vi "laserDiagnose.vi"(0 "405 Port":refnum<visa-resource-name>, 1 "ms to wait (50)":u32=50, 5 "532 Port":refnum<visa-resource-name>, 7 "660 Port":refnum<visa-resource-name>, 9 "785 Port":refnum<visa-resource-name>, 11 "error in (no error)":errorcluster) -> (4 "Currents":T1, 6 "Temperatures":T2, 10 "Powers":T3, 14 "Overtemp":bool, 15 "error out":errorcluster)   [LabVIEW 2011]
panel:
  out "660 Port Out":refnum<visa-resource-name>
  out "532 Port Out":refnum<visa-resource-name>
  out "405 Port Out":refnum<visa-resource-name>
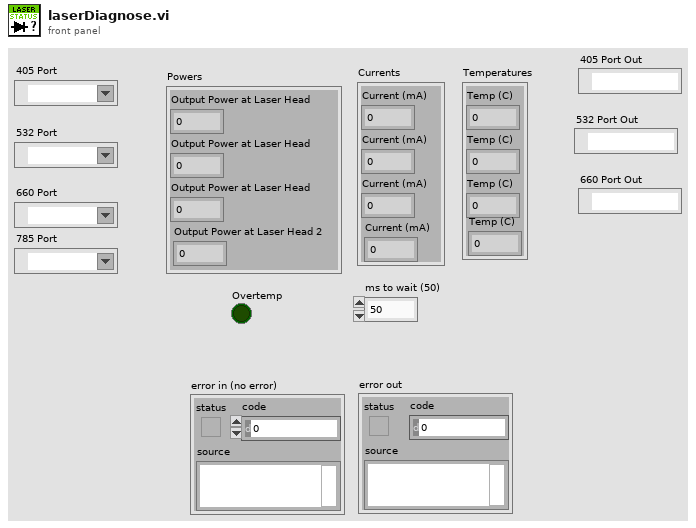
[diagram p1: front panel]
types:
  T1 = cluster{"Current (mA)":dbl, "Current (mA)":dbl, "Current (mA)":dbl, "Current (mA)":dbl}
  T2 = cluster{"Temp (C)":dbl, "Temp (C)":dbl, "Temp (C)":dbl, "Temp (C)":dbl}
  T3 = cluster{"Output Power at Laser Head":dbl, "Output Power at Laser Head":dbl, "Output Power at Laser Head":dbl, "Output Power at Laser Head 2":dbl}
  T4 = cluster{"Current, mA":dbl, "Current, mA":dbl, "Current, mA":dbl, "Current, mA":dbl}
  T5 = cluster{"Power, mW":dbl, "Power, mW":dbl, "Power, mW":dbl, "Power, mW":dbl}
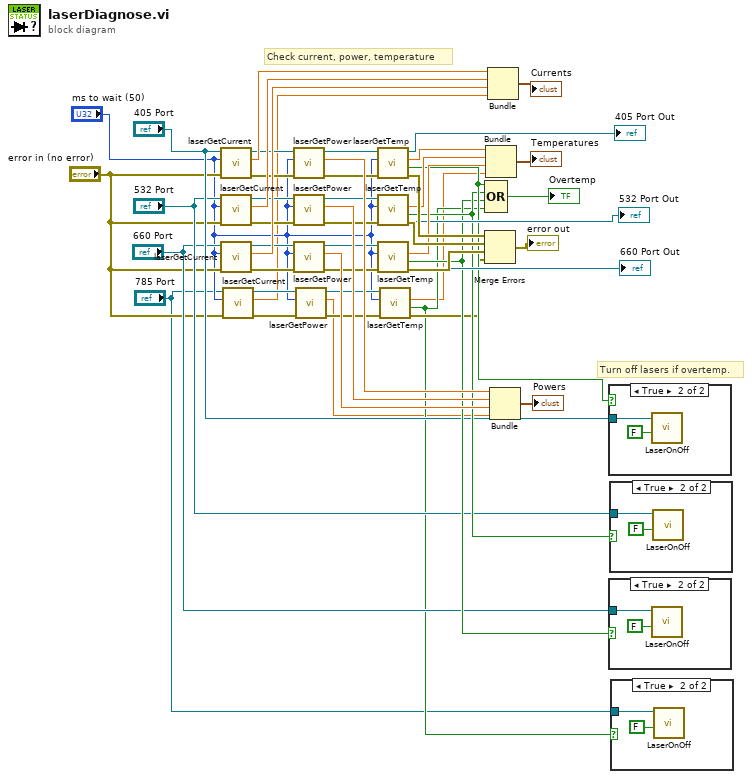
[diagram p0: block diagram]
diagram:
  # "Check current, power, temperature"
  # "Turn off lasers if overtemp."
  n1 = call "laserGetCurrent.vi"("error in (no error)"="error in (no error)", "ms to wait (5)"="ms to wait (50)", "VISA resource name"="405 Port") -> ("error out"=w31:errorcluster, "Current, mA"=w37:dbl, "VISA resource name out"=w25:refnum<visa-resource-name>)  [unwired: 6 in]
  n2 = call "laserGetCurrent.vi"("error in (no error)"="error in (no error)", "ms to wait (5)"="ms to wait (50)", "VISA resource name"="532 Port") -> ("error out"=w33:errorcluster, "Current, mA"=w38:dbl, "VISA resource name out"=w27:refnum<visa-resource-name>)  [unwired: 6 in]
  n3 = call "laserGetCurrent.vi"("error in (no error)"="error in (no error)", "ms to wait (5)"="ms to wait (50)", "VISA resource name"="660 Port") -> ("error out"=w36:errorcluster, "Current, mA"=w39:dbl, "VISA resource name out"=w29:refnum<visa-resource-name>)  [unwired: 6 in]
  n4 = call "laserGetCurrent.vi"("error in (no error)"="error in (no error)", "ms to wait (5)"="ms to wait (50)", "VISA resource name"="785 Port") -> ("error out"=w11:errorcluster, "Current, mA"=w3:dbl, "VISA resource name out"=w14:refnum<visa-resource-name>)  [unwired: 6 in]
  n5 = call "laserGetPower.vi"("error in (no error)"=w31, "ms to wait (5)"="ms to wait (50)", "VISA resource name"=w25) -> ("error out"=w32:errorcluster, "Power, mW"=w43:dbl, "VISA resource name out"=w26:refnum<visa-resource-name>)  [unwired: 6 in]
  n6 = call "laserGetPower.vi"("error in (no error)"=w33, "ms to wait (5)"="ms to wait (50)", "VISA resource name"=w27) -> ("error out"=w34:errorcluster, "Power, mW"=w44:dbl, "VISA resource name out"=w28:refnum<visa-resource-name>)  [unwired: 6 in]
  n7 = call "laserGetPower.vi"("error in (no error)"=w36, "ms to wait (5)"="ms to wait (50)", "VISA resource name"=w29) -> ("error out"=w35:errorcluster, "Power, mW"=w45:dbl, "VISA resource name out"=w30:refnum<visa-resource-name>)  [unwired: 6 in]
  n8 = call "laserGetPower.vi"("error in (no error)"=w11, "ms to wait (5)"="ms to wait (50)", "VISA resource name"=w14) -> ("error out"=w12:errorcluster, "Power, mW"=w2:dbl, "VISA resource name out"=w13:refnum<visa-resource-name>)  [unwired: 6 in]
  n9 = call "laserGetTemp.vi"("error in (no error)"=w32, "milliseconds to wait"="ms to wait (50)", "VISA resource name"=w26) -> ("error out"=w47:errorcluster, "Overtemp"=w20:bool, "Temp (C)"=w5:dbl, "VISA resource name out"=→"405 Port Out":refnum<visa-resource-name>)  [unwired: 5 in]
  n10 = call "laserGetTemp.vi"("error in (no error)"=w34, "milliseconds to wait"="ms to wait (50)", "VISA resource name"=w28) -> ("error out"=w48:errorcluster, "Overtemp"=w19:bool, "Temp (C)"=w41:dbl, "VISA resource name out"=→"532 Port Out":refnum<visa-resource-name>)  [unwired: 5 in]
  n11 = call "laserGetTemp.vi"("error in (no error)"=w35, "milliseconds to wait"="ms to wait (50)", "VISA resource name"=w30) -> ("error out"=w49:errorcluster, "Overtemp"=w18:bool, "Temp (C)"=w42:dbl, "VISA resource name out"=→"660 Port Out":refnum<visa-resource-name>)  [unwired: 5 in]
  n12 = call "laserGetTemp.vi"("error in (no error)"=w12, "milliseconds to wait"="ms to wait (50)", "VISA resource name"=w13) -> ("error out"=w10:errorcluster, "Overtemp"=w9:bool, "Temp (C)"=w6:dbl)  [unwired: 5 in, 1 out]
  n13 = Compound Arithmetic op=OR(w20, w19, w18, w9) -> (→"Overtemp":bool)
  n14 = Merge Errors(w47, w48, w49, w10) -> (→"error out":errorcluster)
  n15 = Bundle("Temp (C)"=w5, "Temp (C)"=w41, "Temp (C)"=w42, "Temp (C)"=w6) -> (→"Temperatures":T2)  [unwired: 1 in]
  n16 = Bundle("Current, mA"=w37, "Current, mA"=w38, "Current, mA"=w39, "Current, mA"=w3) -> (→"Currents":T4)  [unwired: 1 in]
  n17 = Bundle("Power, mW"=w43, "Power, mW"=w44, "Power, mW"=w45, "Power, mW"=w2) -> (→"Powers":T5)  [unwired: 1 in]
  n18 = case shown="True" w20 {
    tunnel: "405 Port" -> [_ w52]
    frame False {
    }
    frame True {
      n19 = call "LaserOnOff.vi"("Emission (F = OFF)"=FALSE ("405 Emission (T = ON)"), "VISA Refnum in"=w52) -> ()  [unwired: 7 in, 3 out]
    }
  }
  n20 = case shown="True" w18 {
    tunnel: "660 Port" -> [_ w54]
    frame False {
    }
    frame True {
      n21 = call "LaserOnOff.vi"("Emission (F = OFF)"=FALSE ("405 Emission (T = ON)"), "VISA Refnum in"=w54) -> ()  [unwired: 7 in, 3 out]
    }
  }
  n22 = case shown="True" w19 {
    tunnel: "532 Port" -> [_ w56]
    frame False {
    }
    frame True {
      n23 = call "LaserOnOff.vi"("Emission (F = OFF)"=FALSE ("405 Emission (T = ON)"), "VISA Refnum in"=w56) -> ()  [unwired: 7 in, 3 out]
    }
  }
  n24 = case shown="True" w9 {
    tunnel: "785 Port" -> [_ w58]
    frame False {
    }
    frame True {
      n25 = call "LaserOnOff.vi"("Emission (F = OFF)"=FALSE ("405 Emission (T = ON)"), "VISA Refnum in"=w58) -> ()  [unwired: 7 in, 3 out]
    }
  }
